vi "Serialize.vi"(8 "error in (no error)":errorcluster, 11 "ConverterBase in":refnum<class "FileConverterBase.lvclass">) -> (0 "error out":errorcluster, 2 "JSON":string, 3 "ConverterBase out":refnum<class "FileConverterBase.lvclass">)   [LabVIEW 2017, in "FileConverterBase.lvclass"]
uses:
  FileConverterBase.lvclass
  JSONConstants.vi
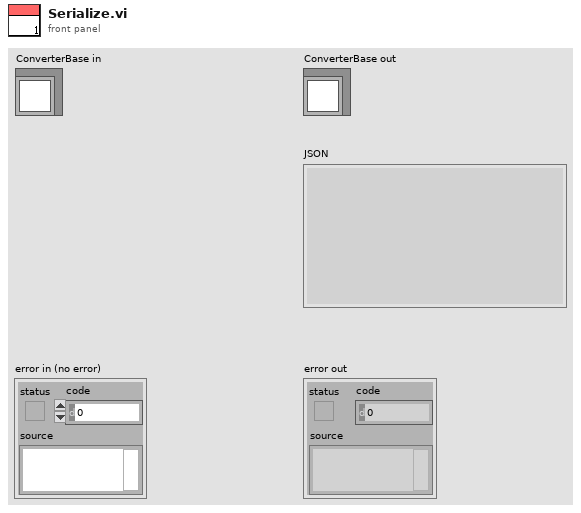
[diagram p1: front panel]
types:
  T1 = typedef "SupportedFileTypes.ctl" = enum16{"VirtualInstrument", "Polymorphic VI", "Class", "Project"}
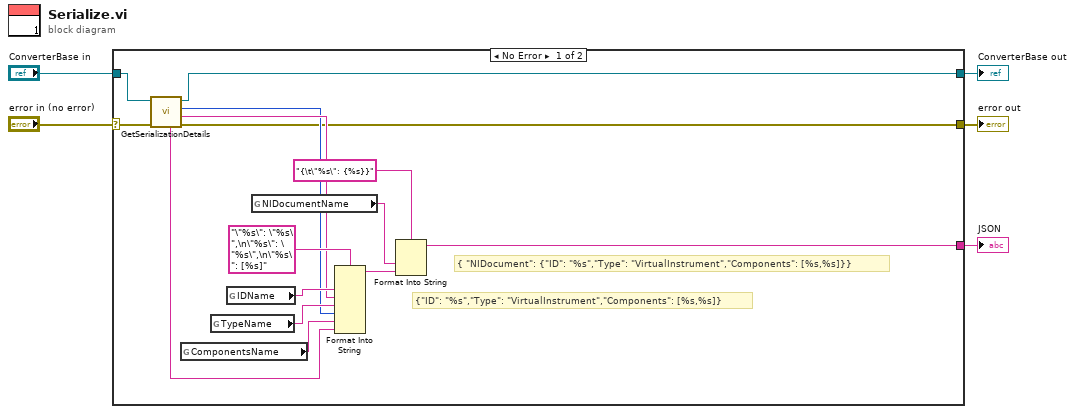
[diagram p0: block diagram]
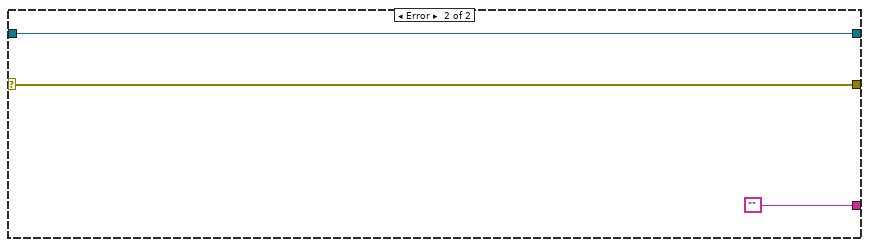
[diagram p2: hidden frame]
diagram:
  n1 = case shown="No Error" "error in (no error)" {
    selector: "error in (no error)" -> [w8 w23]
    tunnel: [w7 w23] -> w4
    tunnel: [w9 w22] -> w2
    tunnel: "ConverterBase in" -> [w10 w22]
    tunnel: [w6 ""] -> w1
    frame No Error {
      # "{\t\"NIDocument\": {\"ID\": \"%s\",\"Type\": \"VirtualInstrument\",\"Components\": [%s,%s]}}"
      # "{\"ID\": \"%s\",\"Type\": \"VirtualInstrument\",\"Components\": [%s,%s]}"
      n2 = call-dynamic "GetSerializationDetails.vi"("error in (no error)"=w8, "FileConverterBase in"=w10) -> ("error out"=w7:errorcluster, "ID"=w12:string, "FileType"=w11:T1, "FileConverterBase out"=w9:refnum<class "FileConverterBase.lvclass">, "ComponentsSerialized"=w13:string)  [unwired: 5 in]
      n3 = global read "JSONConstants.vi" "ComponentsName"() -> (w20:string)
      n4 = global read "JSONConstants.vi" "TypeName"() -> (w19:string)
      n5 = global read "JSONConstants.vi" "IDName"() -> (w18:string)
      n6 = global read "JSONConstants.vi" "NIDocumentName"() -> (w15:string)
      n7 = Format Into String(format string="\"%s\": \"%s\",\n\"%s\": \"%s\",\n\"%s\": [%s]", w18, w12, w19, w11, w20, w13) -> (resulting string=w17:string)  [unwired: 2 in, 1 out]
      n8 = Format Into String(format string="{\t\"%s\": {%s}}", w15, w17) -> (resulting string=w6:string)  [unwired: 2 in, 1 out]
    }
    frame Error {
    }
  }
  "error out" <- w4
  "ConverterBase out" <- w2
  "JSON" <- w1
